vi "ArmController.vi"(8 "Down":bool, 9 "Up":bool, 10 "Vertical Control":bool, 11 "Horizontal Control":bool) -> (1 "Setpoint":i32, 2 "Horz/Vert":bool)   [LabVIEW 2014]
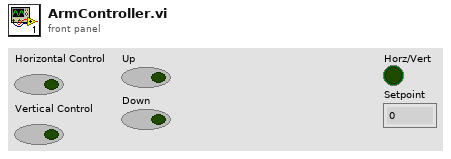
[diagram p1: front panel]
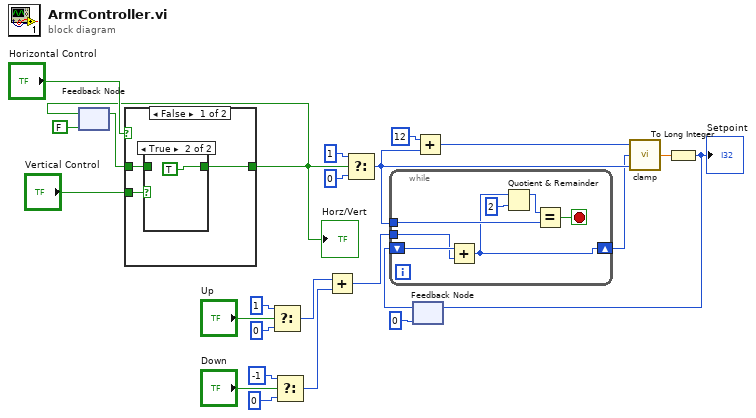
[diagram p0: block diagram]
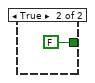
[diagram p3: hidden frame]
diagram:
  n1 = feedback #1(FALSE) -> (w19:bool)
  n2 = case shown="False" "Horizontal Control" {
    tunnel: "Vertical Control" -> [w25 _]
    tunnel: w19 -> [w27 _]
    tunnel: [w26 FALSE] -> w18
    frame False {
      n3 = case shown="True" w25 {
        tunnel: w27 -> [w28 _]
        tunnel: [w28 TRUE] -> w26
        frame False {
        }
        frame True {
        }
      }
    }
    frame True {
    }
  }
  "Horz/Vert" <- w18
  n4 = feedback-in #1(w18) -> ()
  n5 = Select(t=1, s="Up", f=0) -> (s? t:f=w8:i32)
  n6 = Select(t=-1, s="Down", f=0) -> (s? t:f=w9:i32)
  n7 = Add(x=w8, y=w9) -> (x+y=w7:i32)
  n8 = Select(t=1, s=w18, f=0) -> (s? t:f=w4:i32)
  n9 = feedback #2(0) -> (w16:i32)
  n10 = while {
    shift-right: [w33] -> w3
    shift-left: w16 -> [w37]
    tunnel: w7 -> [w36]
    tunnel: w4 -> [w35]
    stop <- w34 stop-if-true
    n11 = Add(x=w37, y=w36) -> (x+y=w33:i32)
    n12 = Quotient & Remainder(x=w33, y=2) -> (x-y*floor(x/y)=w31:i32)  [unwired: 1 out]
    n13 = Equal?(x=w31, y=w35) -> (x = y?=w34:bool)
  }
  n14 = Add(x=12, y=w4) -> (x+y=w5:i32)
  n15 = call "clamp.vi"("Min"=w4, "Input"=w3, "Max"=w5) -> ("Output"=w2:dbl)
  n16 = To Long Integer(number=w2) -> (32bit integer=w1:i32)
  "Setpoint" <- w1
  n17 = feedback-in #2(w1) -> ()
